vi "Create Dataset 3D Double.vi"(7 "Chunk size":u64, 8 "error in (no error)":errorcluster, 9 "Datatype":dbl[][][](array[numeric]), 10 "Dataset name":string, 11 "Locaiton id in":i32) -> (0 "error out":errorcluster, 3 "Datset id":i32)   [LabVIEW 2011]
uses:
  Release/HDF5Tools.dll
  HDF5Tools.lvlib
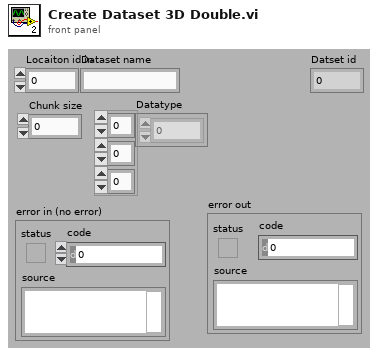
[diagram p1: front panel]
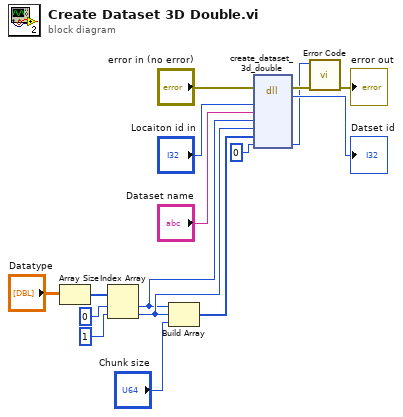
[diagram p0: block diagram]
diagram:
  n1 = Array Size(array="Datatype") -> (size(s)=w8:i32[])
  n2 = Index Array(array=w8, index #1=0 ("index"), index #2=1 ("index")) -> (element #1=w1:i32, element #2=w2:i32)
  n3 = Build Array(w1, w2, "Chunk size") -> (w3:u64[])
  n4 = dll-call lib="F:/HDF5Tools/Release/HDF5Tools.dll" fn="create_dataset_3d_double"(error in="error in (no error)", "loc_id"="Locaiton id in", "name"="Dataset name", "dim1"=w1, "dim2"=w2, "chunks"=w3, "error"=0) -> (error out=w12:errorcluster, "dataset_id"=→"Datset id":i32, "error"=w10:i32)  [unwired: 7 in, 1 out]
  n5 = call "Error Code.vi"("Error in"=w12, "Error code"=w10) -> ("Error out"=→"error out":errorcluster)  [unwired: 9 in]
